vi "Focus Maximal Value.vi"(0 "Gantry In":refnum<k24>, 3 "error in":errorcluster) -> (6 "Gantry Out":refnum<k24>, 9 "error out":errorcluster)   [LabVIEW 2021, in "Component Tray.lvclass"]
uses:
  Component/Component Tray.lvclass
  C:/Program Files (x86)/Aerotech/A3200/LabVIEW/2010/Bin/Aerotech.A3200.dll
  Program Files (x86)/Aerotech/A3200/LabVIEW/2010/Bin/Aerotech.A3200.dll
  Controller/Motion/A3200/A3200.lvclass
  <vilib>/Analysis/NI_AALBase.lvlib
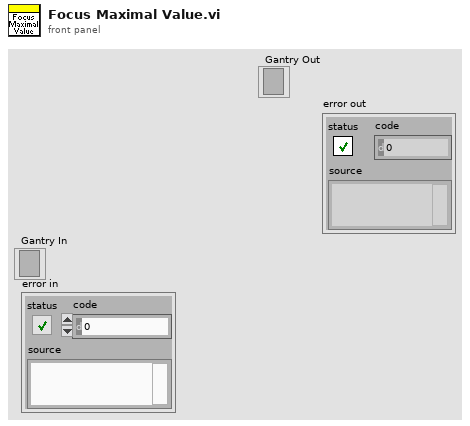
[diagram p1: front panel]
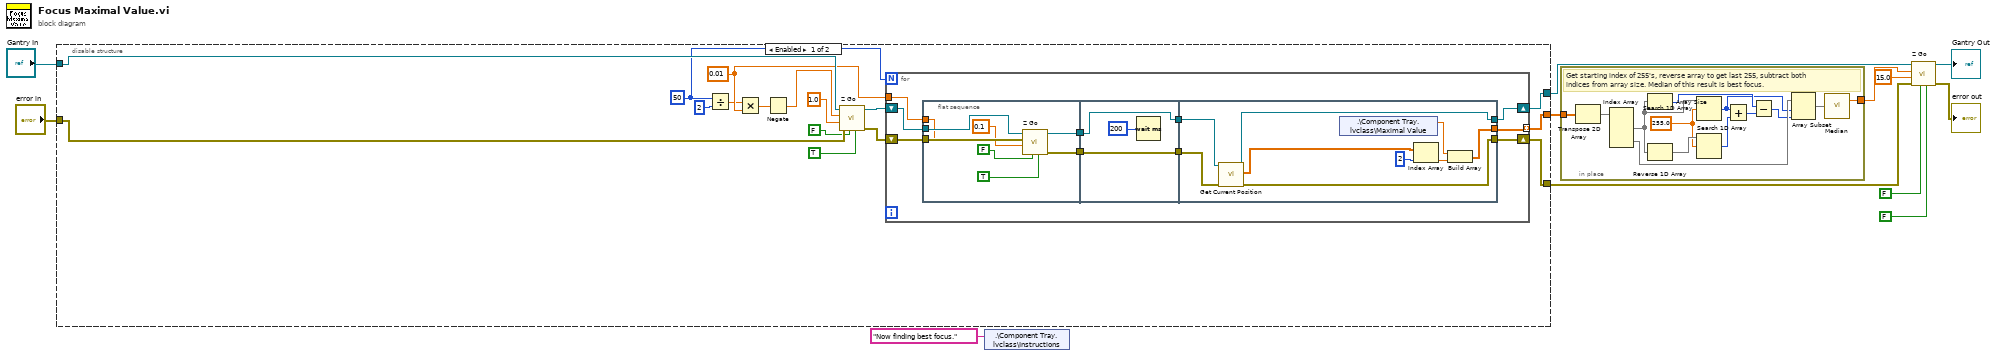
[diagram p0: block diagram]
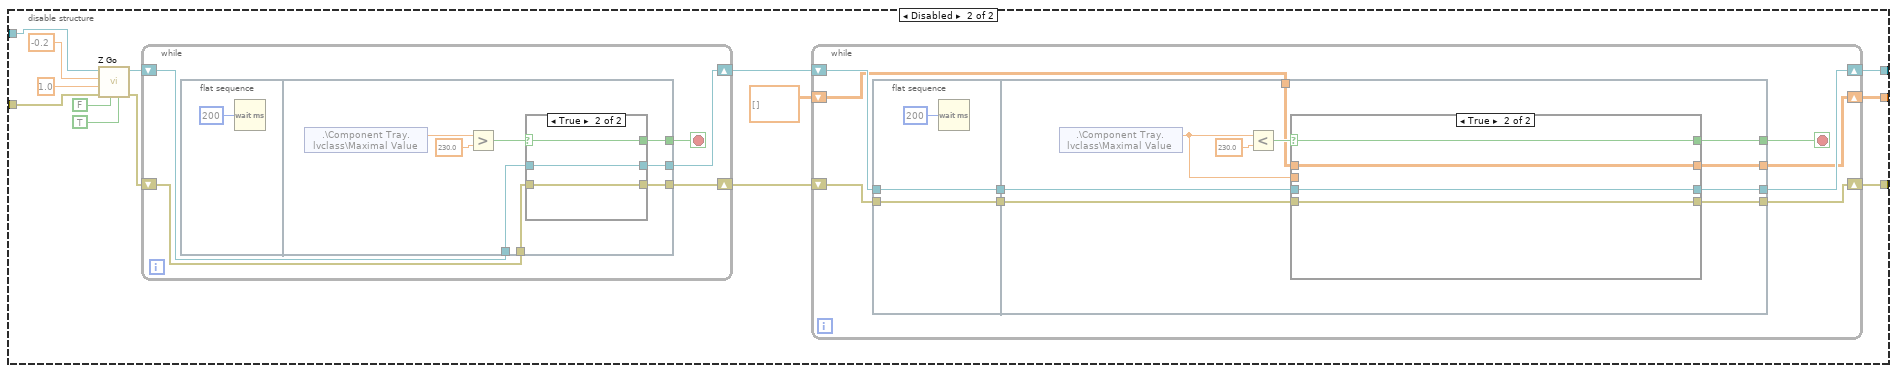
[diagram p2: hidden frame]
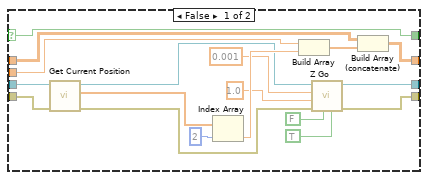
[diagram p3: hidden frame]
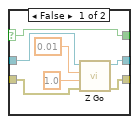
[diagram p4: hidden frame]
diagram:
  n1 = disable-structure shown="Enabled" {
    disable-tunnel: "Gantry In" -> [w28 w72]
    disable-tunnel: "error in" -> [w27 w71]
    disable-tunnel: [w25 w61] -> w9
    disable-tunnel: [w24 w59] -> w8
    disable-tunnel: [w13 w60] -> w3
    frame Enabled {
      w26 = 0.01 ("Focus step size")
      w14 = 50 ("number of focus steps")
      n2 = Divide(x=w14, y=2) -> (x/y=w22:dbl)
      n3 = Multiply(x=w22, y=w26) -> (x*y=w21:dbl)
      n4 = Negate(x=w21) -> (-x=w19:dbl)
      n5 = call "Z Go.vi"("Increment"=TRUE, "Return Immediately"=FALSE ("Increment"), "error in (no error)"=w27, "Speed In"=1.0 ("Speed"), "Position In"=w19, "Gantry In"=w28) -> ("error out"=w17:errorcluster, "Gantry Out"=w18:refnum<k24>)  [unwired: 2 in, 2 out]
      n6 = for {
        N: w14 -> [_]
        tunnel: [w36] -> w13 mode=indexing
        shift-right: [w37] -> w25
        shift-left: w18 -> [w38]
        tunnel: w26 -> [w29]
        shift-right: [w34] -> w24
        shift-left: w17 -> [w35]
        n7 = flat-sequence {
          tunnel: w38 -> [w46]
          tunnel: [w45] -> w33
          tunnel: w35 -> [w44]
          tunnel: [w43] -> w31
          tunnel: w29 -> [w41]
          tunnel: w33 -> [w49]
          tunnel: [w49] -> w32
          tunnel: w31 -> [w48]
          tunnel: [w48] -> w30
          tunnel: w32 -> [w58]
          tunnel: [w57] -> w37
          tunnel: [w56] -> w36
          tunnel: w30 -> [w55]
          tunnel: [w54] -> w34
          frame #0 {
            n8 = call "Z Go.vi"("Increment"=TRUE, "Return Immediately"=FALSE ("Increment"), "error in (no error)"=w44, "Speed In"=0.1 ("Speed"), "Position In"=w41, "Gantry In"=w46) -> ("error out"=w43:errorcluster, "Gantry Out"=w45:refnum<k24>)  [unwired: 2 in, 2 out]
          }
          frame #1 {
            n9 = Wait (ms)(milliseconds to wait=u32 200) -> ()  [unwired: 1 out]
          }
          frame #2 {
            n10 = call "Get Current Position.vi"("error in (no error)"=w55, "Gantry In"=w58) -> ("error out"=w54:errorcluster, "XYZTheta Out"=w53:dbl[], "Gantry Out"=w57:refnum<k24>)  [unwired: 7 in]
            n11 = shared-variable ".\\Component Tray.lvclass\\Maximal Value"() -> (w51:sgl)  [unwired: 1 in, 1 out]
            n12 = Index Array(array=w53, index=2) -> (element=w50:dbl)
            n13 = Build Array(w51, w50) -> (w56:dbl[])
          }
        }
      }
    }
    frame Disabled {
      n14 = call "Z Go.vi"("Increment"=TRUE, "Return Immediately"=FALSE, "error in (no error)"=w71, "Speed In"=1.0, "Position In"=-0.2, "Gantry In"=w72) -> ("error out"=w65:errorcluster, "Gantry Out"=w66:refnum<k24>)  [unwired: 2 in, 2 out]
      n15 = while {
        shift-right: [w118] -> w64
        shift-left: w66 -> [w120]
        shift-right: [w117] -> w63
        shift-left: w65 -> [w119]
        stop <- w121 stop-if-true
        n16 = flat-sequence {
          tunnel: [w128] -> w121
          tunnel: w120 -> [w127]
          tunnel: w119 -> [w126]
          tunnel: [w124] -> w118
          tunnel: [w123] -> w117
          frame #0 {
            n17 = Wait (ms)(milliseconds to wait=u32 200) -> ()  [unwired: 1 out]
          }
          frame #1 {
            n18 = shared-variable ".\\Component Tray.lvclass\\Maximal Value"() -> (w129:sgl)  [unwired: 1 in, 1 out]
            n19 = Greater?(x=w129, y=sgl 230.0) -> (0:w130:bool)
            n20 = case shown="True" w130 {
              selector: w130 -> [w133 w140]
              tunnel: [w133 w140] -> w128
              tunnel: w127 -> [w137 w139]
              tunnel: w126 -> [w136 w138]
              tunnel: [w132 w139] -> w124
              tunnel: [w131 w138] -> w123
              frame False {
                n21 = call "Z Go.vi"("error in (no error)"=w136, "Speed In"=1.0, "Position In"=0.01, "Gantry In"=w137) -> ("error out"=w131:errorcluster, "Gantry Out"=w132:refnum<k24>)  [unwired: 4 in, 2 out]
              }
              frame True {
              }
            }
          }
        }
      }
      n22 = while {
        shift-right: [w80] -> w61
        shift-left: w64 -> [w81]
        shift-right: [w77] -> w59
        shift-left: w63 -> [w78]
        shift-right: [w79] -> w60
        shift-left: dbl[][] [] -> [w73]
        stop <- w74 stop-if-true
        n23 = flat-sequence {
          tunnel: [w84] -> w76
          tunnel: [w83] -> w75
          tunnel: w81 -> [w84]
          tunnel: w78 -> [w83]
          tunnel: w76 -> [w87]
          tunnel: [w88] -> w80
          tunnel: [w90] -> w79
          tunnel: w75 -> [w86]
          tunnel: [w89] -> w77
          tunnel: [w92] -> w74
          tunnel: w73 -> [w85]
          frame #0 {
            n24 = Wait (ms)(milliseconds to wait=u32 200) -> ()  [unwired: 1 out]
          }
          frame #1 {
            n25 = shared-variable ".\\Component Tray.lvclass\\Maximal Value"() -> (w91:sgl)  [unwired: 1 in, 1 out]
            n26 = Less?(x=w91, y=sgl 230.0) -> (x < y?=w93:bool)
            n27 = case shown="True" w93 {
              selector: w93 -> [w112 w116]
              tunnel: [w112 w116] -> w92
              tunnel: w91 -> [w108 _]
              tunnel: [w99 w113] -> w90
              tunnel: [w102 w115] -> w89
              tunnel: [w105 w114] -> w88
              tunnel: w87 -> [w107 w114]
              tunnel: w86 -> [w104 w115]
              tunnel: w85 -> [w101 w113]
              frame False {
                n28 = call "Get Current Position.vi"("error in (no error)"=w104, "Gantry In"=w107) -> ("error out"=w103:errorcluster, "XYZTheta Out"=w110:dbl[], "Gantry Out"=w106:refnum<k24>)  [unwired: 7 in]
                n29 = Index Array(array=w110, index=2) -> (element=w111:dbl)
                n30 = Build Array(w108, w111) -> (w100:dbl[])
                n31 = call "Z Go.vi"("Increment"=TRUE, "Return Immediately"=FALSE, "error in (no error)"=w103, "Speed In"=1.0, "Position In"=0.001, "Gantry In"=w106) -> ("error out"=w102:errorcluster, "Gantry Out"=w105:refnum<k24>)  [unwired: 2 in, 2 out]
                n32 = Build Array (concatenate)(w101, w100) -> (w99:dbl[][])
              }
              frame True {
              }
            }
          }
        }
      }
    }
  }
  n33 = shared-variable ".\\Component Tray.lvclass\\Instructions"("Now finding best focus." ("Instructions")) -> ()  [unwired: 1 in, 1 out]
  n34 = in-place {
    in-place-border: w3 -> [w153]
    in-place-border: [w141] -> w2
    w148 = 255.0 ("element")
    # "Get starting index of 255's, reverse array to get last 255, subtract both indices from array size. Median of this result is best focus."
    n35 = Transpose 2D Array(2D array=w153) -> (transposed array=w152:dbl[][])
    n36 = Index Array(array=w152) -> (element #1=w150:dbl[], element #2=w145:dbl[])  [unwired: 4 in]
    n37 = Array Size(array=w150) -> (size(s)=w151:i32)
    n38 = Reverse 1D Array(array=w150) -> (reversed array=w149:dbl[])
    n39 = Search 1D Array(1D array=w150, element=w148) -> (index of element=w144:i32)  [unwired: 1 in]
    n40 = Search 1D Array(1D array=w149, element=w148) -> (index of element=w146:i32)  [unwired: 1 in]
    n41 = Add(x=w144, y=w146) -> (x+y=w147:i32)
    n42 = Subtract(x=w151, y=w147) -> (x-y=w143:i32)
    n43 = Array Subset(array=w145, index=w144, length=w143) -> (w142:dbl[])
    n44 = call <vilib>:"Median.vi"("X"=w142) -> ("median"=w141:dbl)  [unwired: 1 out]
  }
  n45 = call "Z Go.vi"("Increment"=FALSE, "Return Immediately"=FALSE ("Increment"), "error in (no error)"=w8, "Speed In"=15.0 ("Speed"), "Position In"=w2, "Gantry In"=w9) -> ("error out"=→"error out":errorcluster, "Gantry Out"=→"Gantry Out":refnum<k24>)  [unwired: 2 in, 2 out]
